vi "GuiArduinoLED.vi"() -> ()   [LabVIEW 2011]
uses:
  <vilib>/LabVIEW Interface for Arduino/Type Defs/Pin Mode.ctl
  <vilib>/LabVIEW Interface for Arduino/LabVIEW Interface for Arduino.lvlib
panel:
  out "Debug\nloop count":i32
  in  "LED2 Pin":u8
  in  "LED1 Pin":u8
  in  "LED 2\nduty cycle":u8(knob) step=1 scale=0.0..255.0
  in  "LED 1\nduty cycle":u8(knob) step=1 scale=0.0..255.0
  in  "Stop":bool
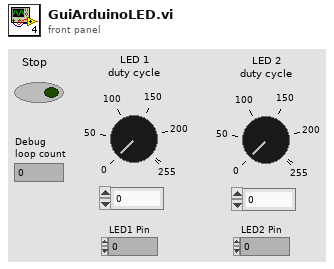
[diagram p1: front panel]
types:
  T1 = typedef "LabVIEW Interface for Arduino.lvlib/Pin Mode.ctl" = enum8{"Input", "Output"}
  T2 = typedef "LabVIEW Interface for Arduino.lvlib/Arduino Resource.ctl" = cluster{"VISA resource":refnum<visa-resource-name>, "Board Type":T3, "Connection Type":enum8{"USB / Serial"}, "Bytes Per Packet (15)":u8}
  T3 = typedef "LabVIEW Interface for Arduino.lvlib/Board Type.ctl" = enum16{"Uno", "Dimuelanove w/Atmega 328", "Mega 2560"}
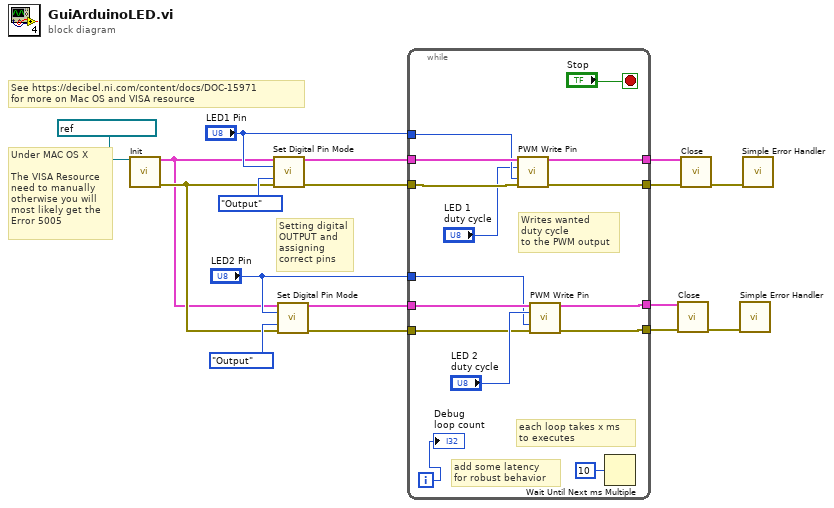
[diagram p0: block diagram]
diagram:
  # "See https://decibel.ni.com/content/docs/DOC-15971\nfor more on Mac OS and VISA resource"
  # "Under MAC OS X\n\nThe VISA Resource\nneed to manually\notherwise you will\nmost likely get the \nError 5005"
  # "Setting digital\nOUTPUT and \nassigning \ncorrect pins"
  n1 = call <vilib>:"Init.vi"("VISA resource"=refnum<visa-resource-name> "ASRL1::INSTR") -> ("Arduino Resource"=w1:T2, "error out"=w2:errorcluster)  [unwired: 17 in]
  n2 = call <vilib>:"Set Digital Pin Mode.vi"("Arduino Resource"=w1, "Digital I/O Pin"="LED1 Pin", "Pin Mode (Input)"=Pin_Mode."Output", "error in"=w2) -> ("Arduino Resource"=w14:T2, "error out"=w13:errorcluster)  [unwired: 10 in]
  n3 = call <vilib>:"Set Digital Pin Mode.vi"("Arduino Resource"=w1, "Digital I/O Pin"="LED2 Pin", "Pin Mode (Input)"=Pin_Mode."Output", "error in"=w2) -> ("Arduino Resource"=w8:T2, "error out"=w7:errorcluster)  [unwired: 10 in]
  n4 = while {
    tunnel: [w32] -> w16
    tunnel: w14 -> [w29]
    tunnel: w13 -> [w30]
    tunnel: [w31] -> w15
    tunnel: "LED1 Pin" -> [w26]
    tunnel: w8 -> [w23]
    tunnel: w7 -> [w22]
    tunnel: "LED2 Pin" -> [w21]
    tunnel: [w20] -> w4
    tunnel: [w19] -> w3
    i -> [w18]
    stop <- "Stop" stop-if-true
    # "Writes wanted\nduty cycle\nto the PWM output"
    # "add some latency\nfor robust behavior"
    # "each loop takes x ms \nto executes"
    n5 = call <vilib>:"PWM Write Pin.vi"("Arduino Resource"=w29, "Duty Cycle (0 - 255)"="LED 1\nduty cycle", "PWM Pin (3)"=w26, "error in"=w30) -> ("Arduino Resource"=w32:T2, "error out"=w31:errorcluster)  [unwired: 10 in]
    n6 = call <vilib>:"PWM Write Pin.vi"("Arduino Resource"=w23, "Duty Cycle (0 - 255)"="LED 2\nduty cycle", "PWM Pin (3)"=w21, "error in"=w22) -> ("Arduino Resource"=w20:T2, "error out"=w19:errorcluster)  [unwired: 10 in]
    n7 = Wait Until Next ms Multiple(millisecond multiple=u32 10) -> ()  [unwired: 1 out]
    "Debug\nloop count" <- w18
  }
  n8 = call <vilib>:"Close.vi"("Arduino Resource"=w4, "error in"=w3) -> ("error out"=w5:errorcluster)  [unwired: 13 in]
  n9 = call <vilib>:"Close.vi"("Arduino Resource"=w16, "error in"=w15) -> ("error out"=w17:errorcluster)  [unwired: 13 in]
  n10 = call <vilib>:"Simple Error Handler.vi"("error in (no error)"=w5) -> ()  [unwired: 4 in, 5 out]
  n11 = call <vilib>:"Simple Error Handler.vi"("error in (no error)"=w17) -> ()  [unwired: 4 in, 5 out]
